vi "Set Output State.vi"(8 "error in (no error)":errorcluster, 10 "Output State":bool, 11 "Water Level in":refnum<class "Water Level.lvclass">) -> (0 "error out":errorcluster, 3 "Water Level out":refnum<class "Water Level.lvclass">)   [LabVIEW 2012, in "Water Level.lvclass"]
uses:
  Water Level.lvclass
  Simulation/Simulation Data_Global.vi
  Simulation/Simulation.lvlib
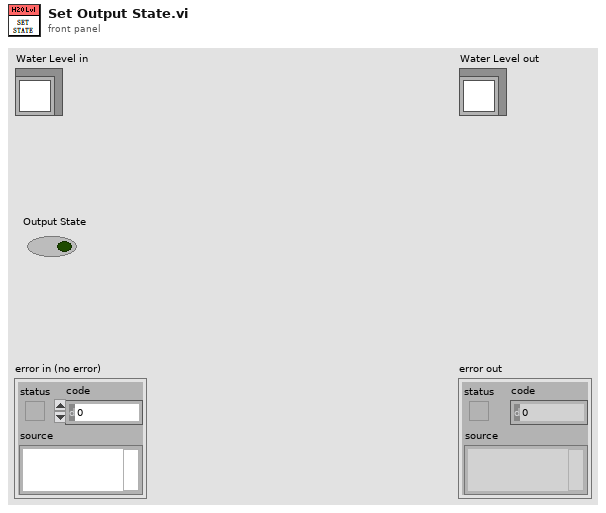
[diagram p1: front panel]
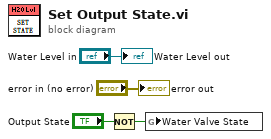
[diagram p0: block diagram]
diagram:
  n1 = Not(x="Output State") -> (.not. x?=w1:bool)
  n2 = global write "Simulation Data_Global.vi" "Water Valve State"(w1) -> ()
  "error out" <- "error in (no error)"
  "Water Level out" <- "Water Level in"
